vi "Initialize-link-unused.vi"(8 "error in (no error)":errorcluster, 11 "Motor-Maxon in":refnum<class "Motor-Xaxis.lvclass">) -> (0 "error out":errorcluster, 3 "Motor-Maxon out":refnum<class "Motor-Xaxis.lvclass">)   [LabVIEW 2013, in "PowderDeposition.lvlib" / "Motor-Xaxis.lvclass"]
uses:
  Motor-Xaxis.lvclass
  Motor-Maxon.lvclass
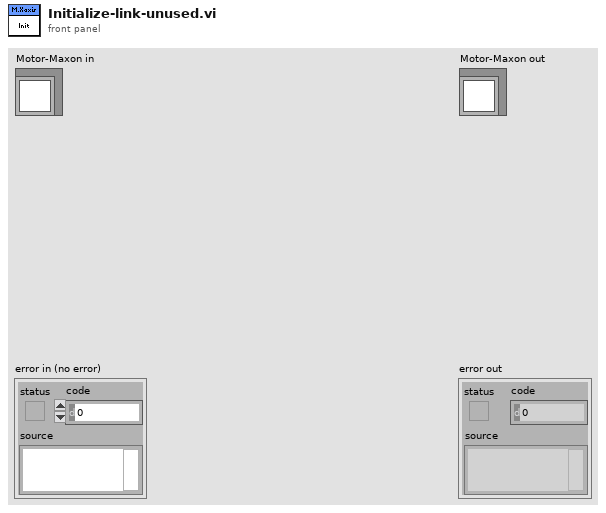
[diagram p1: front panel]
types:
  T1 = cluster{"deviceName":string, "protocolStackName":string, "interfaceName":string, "portName":string, "baudrate":u32, "timeout":u32}
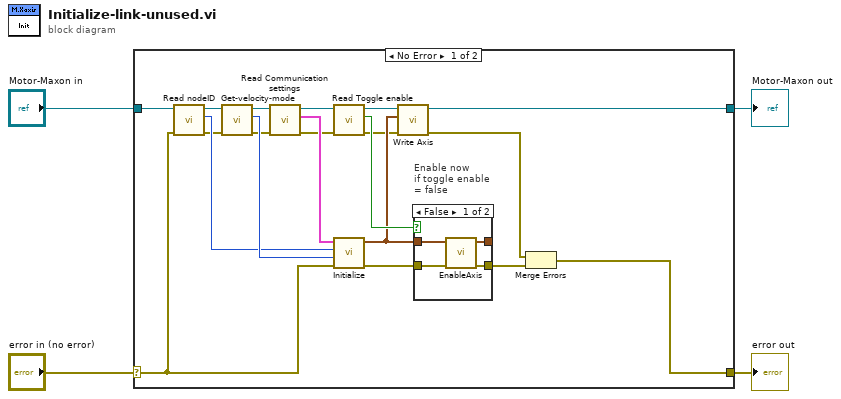
[diagram p0: block diagram]
diagram:
  n1 = case shown="No Error" "error in (no error)" {
    selector: "error in (no error)" -> [w16 w32]
    tunnel: [w15 w32] -> w3
    tunnel: [w6 w31] -> w1
    tunnel: "Motor-Maxon in" -> [w17 w31]
    frame No Error {
      n2 = call-dynamic "Read nodeID.vi"("error in (no error)"=w16, "Motor-Maxon in"=w17) -> ("error out"=w19:errorcluster, "nodeID"=w20:u16, "Motor-Maxon out"=w22:refnum<class "Motor-Xaxis.lvclass">)  [unwired: 7 in]
      n3 = call "Get-velocity-mode.vi"("error in (no error)"=w19, "Motor-Maxon in"=w22) -> ("error out"=w18:errorcluster, "Velocity mode"=w23:i8, "Motor-Maxon out"=w21:refnum<class "Motor-Xaxis.lvclass">)  [unwired: 7 in]
      n4 = call-dynamic "Read Communication settings.vi"("error in (no error)"=w18, "Motor-Maxon in"=w21) -> ("error out"=w13:errorcluster, "Communication settings"=w24:T1, "Motor-Maxon out"=w12:refnum<class "Motor-Xaxis.lvclass">)  [unwired: 7 in]
      n5 = call-dynamic "Read Toggle enable.vi"("error in (no error)"=w13, "Motor-Maxon in"=w12) -> ("error out"=w5:errorcluster, "Toggle enable"=w14:bool, "Motor-Maxon out"=w11:refnum<class "Motor-Xaxis.lvclass">)  [unwired: 7 in]
      n6 = call <instrlib>:"Initialize.vi"("error in (no error)"=w16, "modes of operations"=w23, "nodeId"=w20, "communication settings in"=w24) -> ("error out"=w10:errorcluster, "axis out"=w9:cluster{"keyHandle":u32, "nodeId":u16})  [unwired: 6 in]
      n7 = call-dynamic "Write Axis.vi"("error in (no error)"=w5, "Axis"=w9, "Motor-Maxon in"=w11) -> ("error out"=w7:errorcluster, "Motor-Maxon out"=w6:refnum<class "Motor-Xaxis.lvclass">)  [unwired: 7 in]
      n8 = case "Enable now\nif toggle enable\n= false" shown="False" w14 {
        tunnel: w9 -> [w27 w30]
        tunnel: w10 -> [w28 w29]
        tunnel: [w26 w30] -> _
        tunnel: [w25 w29] -> w8
        frame False {
          n9 = call <instrlib>:"EnableAxis.vi"("error in (no error)"=w28, "axis in"=w27) -> ("error out"=w25:errorcluster, "axis out"=w26:cluster{"keyHandle":u32, "nodeId":u16})  [unwired: 4 in]
        }
        frame True {
        }
      }
      n10 = Merge Errors(w7, w8) -> (w15:errorcluster)
    }
    frame Error {
    }
  }
  "error out" <- w3
  "Motor-Maxon out" <- w1
